vi "unregTcpServerUserEvent.vi"(8 "error in (no error)":errorcluster, 11 "tcpServerBase in":refnum<class "TcpServerBase.lvclass">) -> (0 "error out":errorcluster, 3 "tcpServerBase out":refnum<class "TcpServerBase.lvclass">)   [LabVIEW 2018, in "TcpServerBase.lvclass"]
doc: "Unregister the TcpServer user event. This will be used for TcpServerCmd and TcpServerTelemetry classes."
uses:
  TcpServerBase.lvclass
  TcpServerBase.lvclass/TcpServerBase.ctl
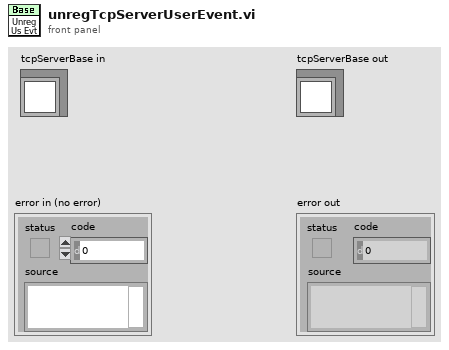
[diagram p1: front panel]
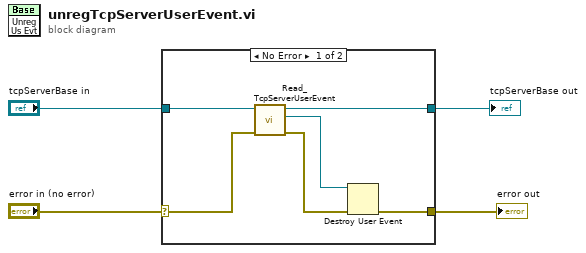
[diagram p0: block diagram]
diagram:
  n1 = case shown="No Error" "error in (no error)" {
    selector: "error in (no error)" -> [w8 w12]
    tunnel: [w7 w12] -> w3
    tunnel: [w9 w11] -> w1
    tunnel: "tcpServerBase in" -> [w10 w11]
    frame No Error {
      n2 = call "Read_TcpServerUserEvent.vi"("error in (no error)"=w8, "TcpServerBase in"=w10) -> ("error out"=w6:errorcluster, "TcpServer"=w5:refnum<user-event>, "TcpServerBase out"=w9:refnum<class "TcpServerBase.lvclass">)  [unwired: 7 in]
      n3 = Destroy User Event(user event=w5, error in=w6) -> (error out=w7:errorcluster)
    }
    frame Error {
    }
  }
  "error out" <- w3
  "tcpServerBase out" <- w1
